vi "target.vi"() -> ()   [LabVIEW 2020]
uses:
  <vilib>/rvi/Emulation/niFpgaGetClockAttributes.vi
  <vilib>/rvi/Emulation/niFpgaSctlEmulationGetInTimedLoop.vi
  <vilib>/rvi/Emulation/niFpgaEmulationReportErrorSimple.vi
  <vilib>/rvi/interface/RandomDataEmulation/niFpgaRandomDataHandleErrors.vi
  <vilib>/rvi/Emulation/niFpgaCriticalErrorInLSC.vi
  <vilib>/rvi/DataTransferAndStorage/Container/XNode/niFpgaContainer.xnode
  <vilib>/rvi/interface/RandomDataEmulation/nirviRandomDataFpgaReadWriteTemplate.vi
  <vilib>/Platform/TimedLoop/XDataNode/wakeup.ctl
  <vilib>/Platform/TimedLoop/XDataNode/XDNodeRunTimeDep.lvlib
  <vilib>/Platform/TimedLoop/XDataNode/nitl_modes.ctl
  <vilib>/Platform/TimedLoop/XDataNode/timing_clust.ctl
  <vilib>/Platform/TimedLoop/XDataNode/XDataNode.xnode
panel:
  out "Timed Out? FIFO out index":bool
  out "Timed Out? FIFO out IMG":bool
  out "Timed Out? FIFO out REAL":bool
  out "Timed Out? FIFO in REAL":bool
  out "Timed Out? FIFO in IMG":bool
  out "sort time (us)":u32
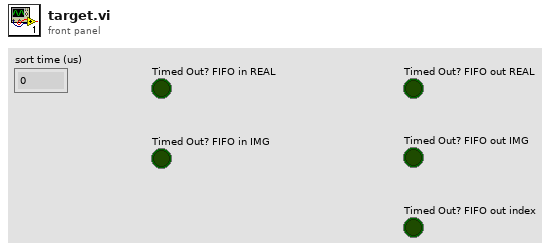
[diagram p1: front panel]
types:
  T1 = typedef "XDNodeRunTimeDep.lvlib/timing_clust.ctl" = cluster{"Expected End [f-1]":u64, "Actual End [f-1]":u64, "Finished Late? [f-1]":bool, "Expected End [i-1]":u64, "Actual End [i-1]":u64, "Finished Late? [i-1]":bool, "Expected Start [i]":u64, "Actual Start [i]":u64, "Expected Start [f]":u64, "Actual Start [f]":u64, "Source Name":string, "Structure Name":string, "Period":i64, "Deadline":i64, "Offset":i64, "Start":i64, "Priority":i32, "Timeout":i32, "Mode":T2, "Wakeup Reason":T3, "Error":errorcluster, "Source Type":string, "Secondary Source Type":string, "Global End Time":u64, "Global Start Time":u64, "Frame Duration":u64, "Iteration Duration":u64, "Assigned CPU":i32, "I/O Scan Engine Mode":u32}
  T2 = typedef "XDNodeRunTimeDep.lvlib/nitl_modes.ctl" = enum32{"No Change", "Process missed periods, maintain original phase", "Discard missed periods, maintain original phase", "Process missed periods, ignore original phase", "Discard missed periods, ignore original phase"}
  T3 = typedef "XDNodeRunTimeDep.lvlib/wakeup.ctl" = enum32{"Normal", "Aborted", "Asynchronous wakeup", "Timing source error", "Timed loop error", "Timeout"}
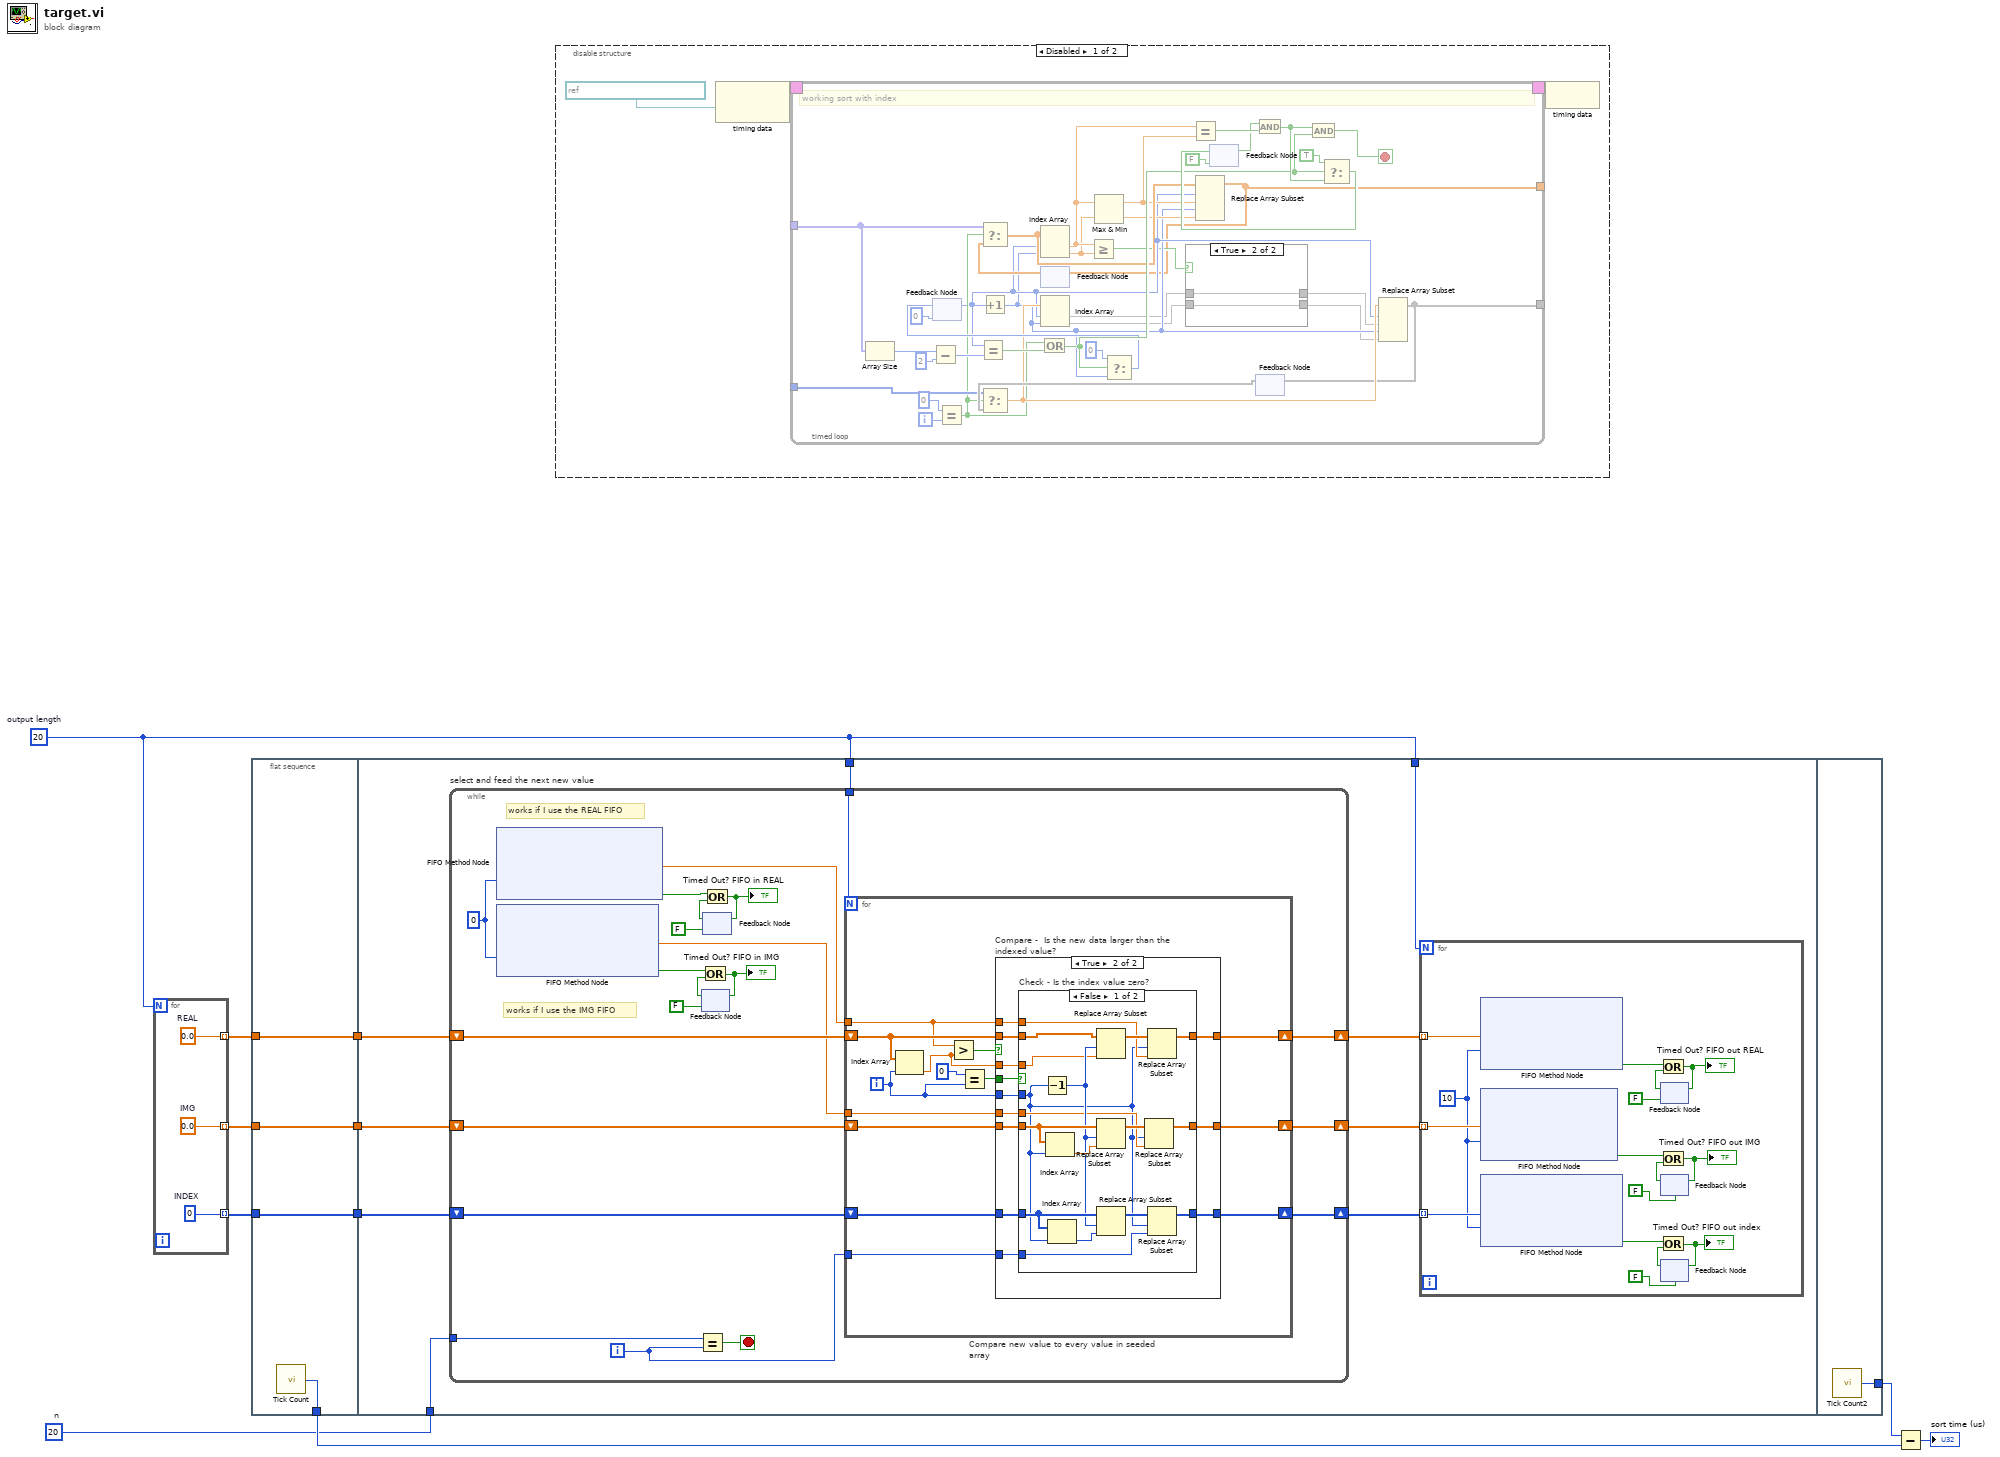
[diagram p0: block diagram]
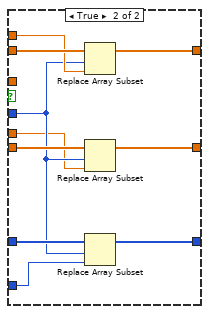
[diagram p5: hidden frame]
diagram:
  w4 = 20  # n
  w3 = 20  # output length
  n1 = for {
    N: w3 -> [_]
    tunnel: [w14] -> w5 mode=indexing
    tunnel: [w13] -> w7 mode=indexing
    tunnel: [w12] -> w1 mode=indexing
    w12 = sgl 0.0  # IMG
    w13 = 0  # INDEX
    w14 = sgl 0.0  # REAL
  }
  n2 = flat-sequence {
    tunnel: [w18] -> w10
    tunnel: [w17] -> w8
    tunnel: w7 -> [w17]
    tunnel: [w16] -> w6
    tunnel: w5 -> [w16]
    tunnel: [w15] -> w2
    tunnel: w1 -> [w15]
    tunnel: w8 -> [w27]
    tunnel: w6 -> [w26]
    tunnel: w4 -> [w24]
    tunnel: w3 -> [w25]
    tunnel: w3 -> [w23]
    tunnel: w2 -> [w19]
    tunnel: [w121] -> w11
    frame #0 {
      n3 = call "Tick Count"() -> ("Tick Count(uSec)"=w18:u32)
    }
    frame #1 {
      n4 = while "select and feed the next new value" {
        shift-right: [w47] -> w21
        shift-left: w26 -> [w48]
        shift-right: [w46] -> w22
        shift-left: w27 -> [w45]
        tunnel: w25 -> [w44]
        tunnel: w24 -> [w42]
        shift-right: [w40] -> w20
        shift-left: w19 -> [w39]
        i -> [w43]
        stop <- w41 stop-if-true
        w38 = 0 ("Timeout")
        # "works if I use the REAL FIFO"
        # "works if I use the IMG FIFO"
        n5 = xnode ("FIFO Method Node")("Timeout"=w38) -> ("Element"=w36:sgl, "Timed Out?"=w28:bool)  [unwired: 1 in, 1 out]
        n6 = xnode ("FIFO Method Node")("Timeout"=w38) -> ("Element"=w37:sgl, "Timed Out?"=w32:bool)  [unwired: 1 in, 1 out]
        n7 = Equal?(x=w42, y=w43) -> (x = y?=w41:bool)
        n8 = feedback #1(FALSE) -> (w33:bool)
        n9 = Or(x=w32, y=w33) -> (x .or. y?=w34:bool)
        "Timed Out? FIFO in IMG" <- w34
        n10 = feedback-in #1(w34) -> ()
        n11 = feedback #2(FALSE) -> (w29:bool)
        n12 = Or(x=w28, y=w29) -> (x .or. y?=w30:bool)
        "Timed Out? FIFO in REAL" <- w30
        n13 = feedback-in #2(w30) -> ()
        n14 = for "Compare new value to every value in seeded array" {
          N: w44 -> [_]
          tunnel: w36 -> [w60]
          shift-right: [w59] -> w47
          shift-left: w48 -> [w61]
          tunnel: w43 -> [w57]
          shift-right: [w55] -> w46
          shift-left: w45 -> [w56]
          shift-right: [w52] -> w40
          shift-left: w39 -> [w51]
          tunnel: w37 -> [w50]
          i -> [w58]
          n15 = Index Array(array=w61, index=w58) -> (element=w49:sgl)
          n16 = Greater?(x=w60, y=w49) -> (0:w62:bool)
          n17 = Equal?(x=0, y=w58) -> (x = y?=w53:bool)
          n18 = case "Compare -  Is the new data larger than the indexed value?" shown="True" w62 {
            tunnel: w61 -> [w65 w76]
            tunnel: w53 -> [_ w77]
            tunnel: w60 -> [_ w75]
            tunnel: w58 -> [_ w74]
            tunnel: [w65 w73] -> w59
            tunnel: w57 -> [_ w72]
            tunnel: w56 -> [w64 w71]
            tunnel: [w64 w70] -> w55
            tunnel: [w63 w69] -> w52
            tunnel: w51 -> [w63 w68]
            tunnel: w50 -> [_ w67]
            tunnel: w49 -> [_ w66]
            frame False {
            }
            frame True {
              n19 = case "Check - Is the index value zero?" shown="False" w77 {
                tunnel: w76 -> [w80 w104]
                tunnel: w75 -> [w93 w103]
                tunnel: w74 -> [w79 w97]
                tunnel: [w92 w102] -> w73
                tunnel: w72 -> [w87 w101]
                tunnel: w71 -> [w89 w100]
                tunnel: [w88 w99] -> w70
                tunnel: [w82 w95] -> w69
                tunnel: w68 -> [w86 w98]
                tunnel: w67 -> [w81 w96]
                tunnel: w66 -> [w78 _]
                frame False {
                  n20 = Decrement(x=w79) -> (x-1=w84:i32)
                  n21 = Index Array(array=w86, index=w79) -> (element=w85:sgl)
                  n22 = Index Array(array=w89, index=w79) -> (element=w91:i32)
                  n23 = Replace Array Subset(array=w80, new element=w78, index=w84) -> (w94:sgl[])
                  n24 = Replace Array Subset(array=w86, new element=w85, index=w84) -> (w83:sgl[])
                  n25 = Replace Array Subset(array=w89, new element=w91, index=w84) -> (w90:i32[])
                  n26 = Replace Array Subset(array=w83, new element=w81, index=w79) -> (w82:sgl[])
                  n27 = Replace Array Subset(array=w94, new element=w93, index=w79) -> (w92:sgl[])
                  n28 = Replace Array Subset(array=w90, new element=w87, index=w79) -> (w88:i32[])
                }
                frame True {
                  n29 = Replace Array Subset(array=w104, new element=w103, index=w97) -> (w102:sgl[])
                  n30 = Replace Array Subset(array=w98, new element=w96, index=w97) -> (w95:sgl[])
                  n31 = Replace Array Subset(array=w100, new element=w101, index=w97) -> (w99:i32[])
                }
              }
            }
          }
        }
      }
      n32 = for {
        N: w23 -> [_]
        tunnel: w22 -> [w120] mode=indexing
        tunnel: w21 -> [w119] mode=indexing
        tunnel: w20 -> [w118] mode=indexing
        w117 = 10 ("Timeout")
        n33 = xnode ("FIFO Method Node")("Element"=w120, "Timeout"=w117) -> ("Timed Out?"=w105:bool)  [unwired: 1 in, 1 out]
        n34 = xnode ("FIFO Method Node")("Element"=w119, "Timeout"=w117) -> ("Timed Out?"=w113:bool)  [unwired: 1 in, 1 out]
        n35 = xnode ("FIFO Method Node")("Element"=w118, "Timeout"=w117) -> ("Timed Out?"=w109:bool)  [unwired: 1 in, 1 out]
        n36 = feedback #3(FALSE) -> (w114:bool)
        n37 = Or(x=w113, y=w114) -> (x .or. y?=w115:bool)
        "Timed Out? FIFO out REAL" <- w115
        n38 = feedback-in #3(w115) -> ()
        n39 = feedback #4(FALSE) -> (w112:bool)
        n40 = Or(x=w109, y=w112) -> (x .or. y?=w111:bool)
        "Timed Out? FIFO out IMG" <- w111
        n41 = feedback-in #4(w111) -> ()
        n42 = feedback #5(FALSE) -> (w108:bool)
        n43 = Or(x=w105, y=w108) -> (x .or. y?=w107:bool)
        "Timed Out? FIFO out index" <- w107
        n44 = feedback-in #5(w107) -> ()
      }
    }
    frame #2 {
      n45 = call "Tick Count2"() -> ("Tick Count(uSec)"=w121:u32)
    }
  }
  n46 = disable-structure shown="Disabled" {
    frame Disabled {
      n47 = node-c288(refnum<k21> "40 MHz Onboard Clock" ("Source Name")) -> (w125:T1)
      n48 = timed-loop {
        tunnel: _ -> [w159]
        tunnel: [w138] -> w123
        timing: w125 -> [_]
        timing-out: [_] -> w124
        tunnel: [w127] -> _
        tunnel: [w126] -> _
        i -> [w142]
        stop <- w143 stop-if-true
        # "working sort with index"
        n49 = Array Size(array=w159) -> (size(s)=w162:i32)
        n50 = Subtract(x=w162, y=2) -> (x-y=w160:i32)
        n51 = feedback #6(0 ("y")) -> (w136:i32)
        n52 = Equal?(x=0, y=w142) -> (x = y?=w137:bool)
        n53 = Equal?(x=w136, y=w160) -> (x = y?=w147:bool)
        n54 = Increment(x=w136) -> (x+1=w135:i32)
        n55 = Or(x=w137, y=w147) -> (x .or. y?=w150:bool)
        n56 = feedback #7() -> (w152:dbl[])  [unwired: 1 in]
        n57 = Select(t=w159, s=w137, f=w152) -> (s? t:f=w146:dbl[])
        n58 = Index Array(array=w146, index #1=w136, index #2=w135) -> (element #1=w130:dbl, element #2=w129:dbl)
        n59 = Greater Or Equal?(x=w130, y=w129) -> (x >= y?=w128:bool)
        n60 = Max & Min(x=w130, y=w129) -> (max(x,y)=w145:dbl, min(x,y)=w144:dbl)
        n61 = Select(t=0 ("y"), s=w150, f=w135) -> (s? t:f=w148:i32)
        n62 = feedback-in #6(w148) -> ()
        n63 = Equal?(x=w130, y=w145) -> (x = y?=w158:bool)
        n64 = Replace Array Subset(array=w146, new element #1=w145, index #1=w136, new element #2=w144, index #2=w135) -> (w127:dbl[])
        n65 = feedback-in #7(w127) -> ()
        n66 = feedback #8(FALSE ("t")) -> (w155:bool)
        n67 = And(x=w155, y=w158) -> (x .and. y?=w153:bool)
        n68 = feedback #9() -> (w140:void[])  [unwired: 1 in]
        n69 = Select(t=w138, s=w137, f=w140) -> (s? t:f=w139:dbl)
        n70 = Index Array(array=w139, index #1=w136, index #2=w135) -> (element #1=w134, element #2=w131)
        n71 = case shown="True" w128 {
          tunnel: w134 -> [w164 w166]
          tunnel: [w163 w166] -> w133
          tunnel: [w164 w165] -> w132
          tunnel: w131 -> [w163 w165]
          frame False {
          }
          frame True {
          }
        }
        n72 = And(x=w153, y=w150) -> (x .and. y?=w143:bool)
        n73 = Select(t=TRUE, s=w150, f=w153) -> (s? t:f=w156:bool)
        n74 = feedback-in #8(w156) -> ()
        n75 = Replace Array Subset(array=w139, new element #1=w133, index #1=w136, new element #2=w132, index #2=w135) -> (w126:void[])
        n76 = feedback-in #9(w126) -> ()
      }
      n77 = node-c288(w124) -> ()
    }
    frame Enabled {
    }
  }
  n78 = Subtract(x=w11, y=w10) -> (x-y=→"sort time (us)":u32)
